vi "Path to String.vi"(11 "Path In":path) -> (3 "Path String":string)   [LabVIEW 2023]
doc: "Converts <b>Path In</b> to <b>Path String</b>. If input path is empty, make output string \"None\"."
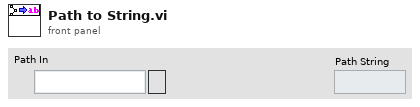
[diagram p1: front panel]
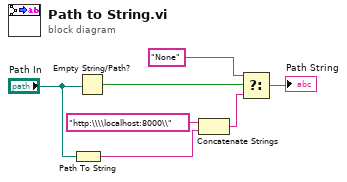
[diagram p0: block diagram]
diagram:
  n1 = Path To String(path="Path In") -> (string=w2:string)
  n2 = Empty String/Path?(string/path="Path In") -> (empty?=w7:bool)
  n3 = Concatenate Strings("http:\\\\localhost:8000\\" ("string"), w2) -> (w1:string)
  n4 = Select(t="None", s=w7, f=w1) -> (s? t:f=→"Path String":string)
